vi "Test Display API.vi"() -> ()   [LabVIEW 2021]
doc: "Display API Tester."
uses:
  Display.lvlib
panel:
  out "ModuleName":string
  in  "Sim?":bool
  in  "Simulation":bool
  in  "Show Block Diagram":bool
  in  "Stop Module":bool
  in  "Start Module":bool
  in  "Hide Module Panel":bool
  in  "Show Module Panel":bool
  out "Status":string
  out "Module Running?":bool
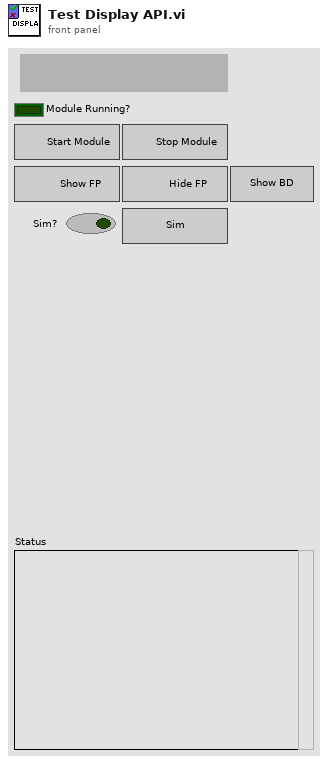
[diagram p1: front panel]
types:
  T1 = typedef "Display.lvlib/Broadcast Events--cluster.ctl" = cluster{"Module Did Init":refnum<user-event>, "Status Updated":refnum<user-event>, "Error Reported":refnum<user-event>, "Module Did Stop":refnum<user-event>, "Update Module Execution Status":refnum<user-event>}
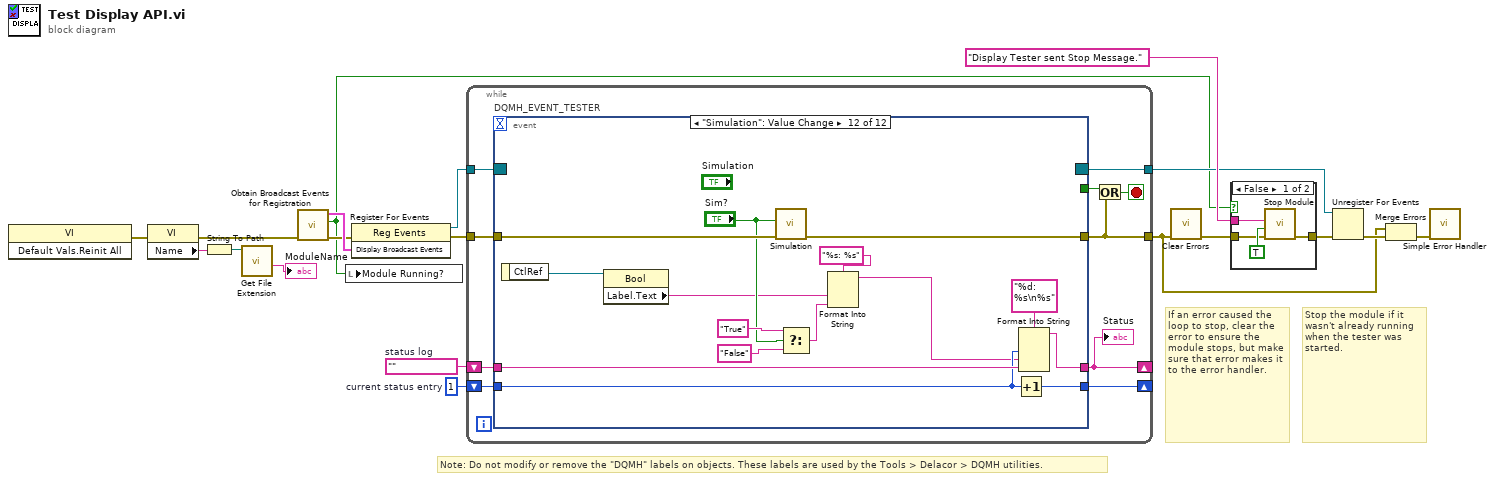
[diagram p0: block diagram]
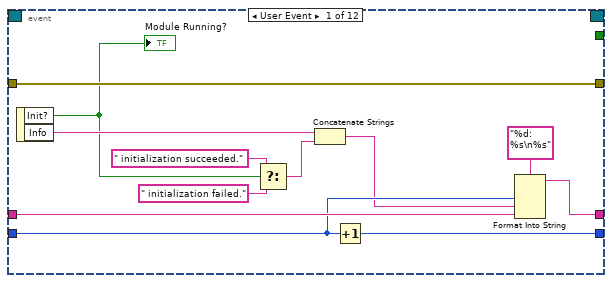
[diagram p3: hidden frame]
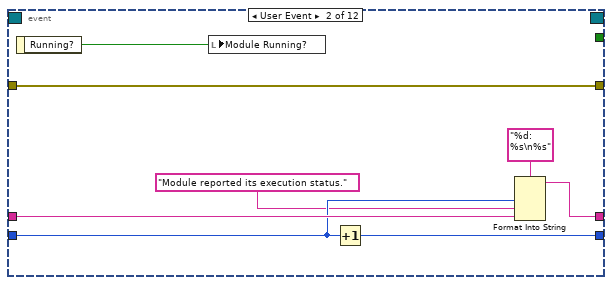
[diagram p4: hidden frame]
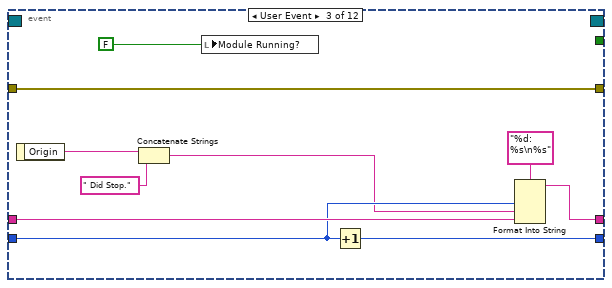
[diagram p5: hidden frame]
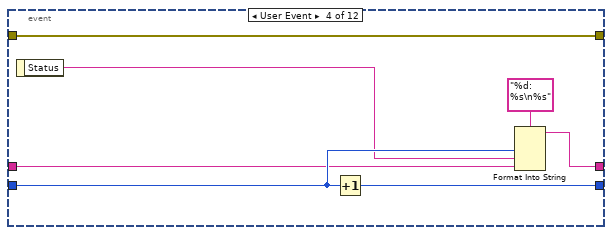
[diagram p6: hidden frame]
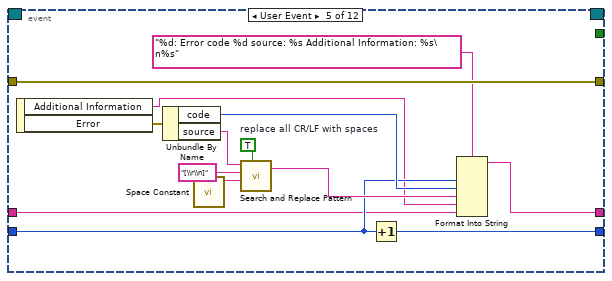
[diagram p7: hidden frame]
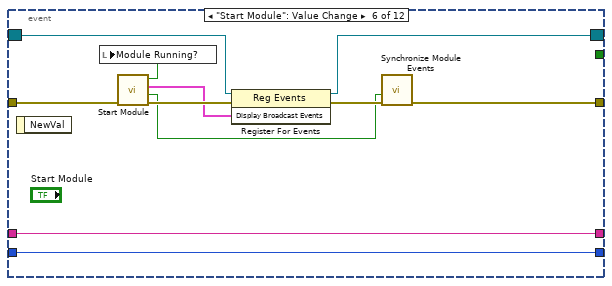
[diagram p8: hidden frame]
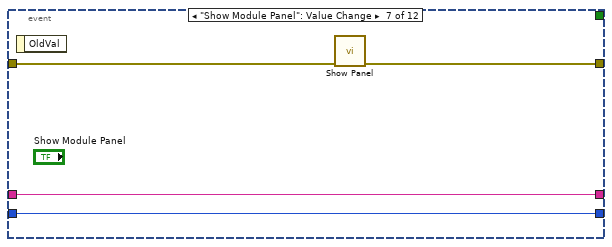
[diagram p9: hidden frame]
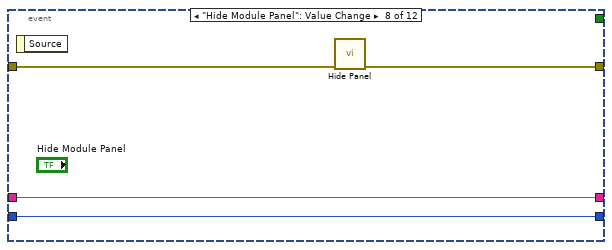
[diagram p10: hidden frame]
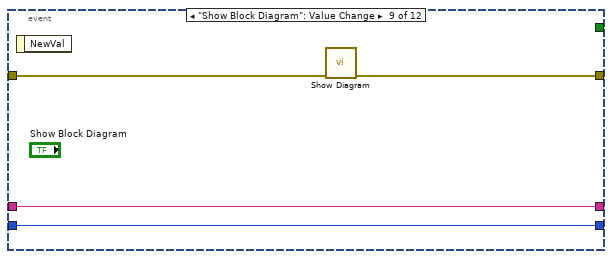
[diagram p11: hidden frame]
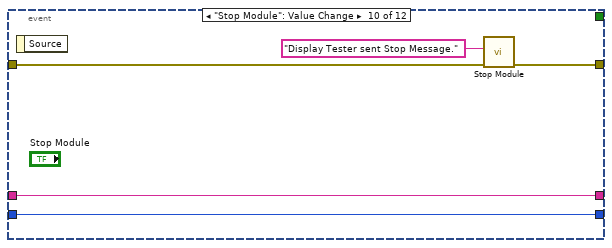
[diagram p12: hidden frame]
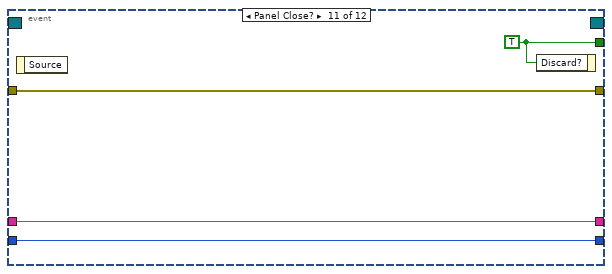
[diagram p13: hidden frame]
diagram:
  w15 = 1  # current status entry
  w16 = ""  # status log
  # "Stop the module if it wasn't already running when the tester was started."
  # "If an error caused the loop to stop, clear the error to ensure the module stops, but make sure that error makes it to the error handler."
  # "Note: Do not modify or remove the \"DQMH\" labels on objects. These labels are used by the Tools > Delacor > DQMH utilities."
  n1 = invoke class="VI" method="Default Vals.Reinit All"() -> (error out=w5:errorcluster)  [unwired: 3 in, 2 out]
  n2 = property class="VI"(error in=w5) -> (error out=w4:errorcluster, "Name"=w2:string)  [unwired: 1 in, 1 out]
  n3 = String To Path(string=w2) -> (path=w1:path)
  n4 = call <vilib>:"Get File Extension.vi"("file"=w1) -> ("filename without extension"=→"ModuleName":string)  [unwired: 6 in, 4 out]
  n5 = call "Obtain Broadcast Events for Registration.vi"("error in (no error)"=w4) -> ("error out"=w7:errorcluster, "Already running?"=w6:bool, "Display Broadcast Events"=w13:T1)  [unwired: 8 in]
  n6 = local write "Module Running?"(w6) -> ()
  n7 = register-events(error in=w7, w13) -> (reference out=w12:refnum<event-registration>, error out=w14:errorcluster)  [unwired: 1 in]
  n8 = while {
    tunnel: w12 -> [w29]
    tunnel: [w20] -> w8
    shift-right: [w24] -> _
    shift-left: w16 -> [w26]
    shift-right: [w25] -> _
    shift-left: w15 -> [w27]
    tunnel: w14 -> [w22]
    tunnel: [w21] -> w11
    stop <- w23 stop-if-true
    n9 = event "DQMH_EVENT_TESTER" shown="[11] \"Simulation\": Value Change" {
      selector: w29 -> [_ _ _ _ _ w85 _ _ _ _ _ _]
      dyn-events: [_ _ _ _ _ w84 _ _ _ _ _ _] -> w21
      timeout: _ -> [_ _ _ _ _ _ _ _ _ _ _ _]
      tunnel: [_ _ _ _ _ _ _ _ _ _ w112 _] -> w28
      tunnel: [w41 w43 w50 w60 w80 w83 w95 w99 w100 w106 w109 w126] -> w20
      tunnel: w27 -> [w38 w47 w57 w63 w70 w88 w93 w97 w101 w107 w110 w121]
      tunnel: w26 -> [w39 w48 w58 w62 w68 w89 w94 w98 w102 w108 w111 w124]
      tunnel: [w36 w45 w55 w64 w71 w89 w94 w98 w102 w108 w111 w123] -> w24
      tunnel: [w37 w46 w56 w66 w69 w88 w93 w97 w101 w107 w110 w122] -> w25
      tunnel: w22 -> [w41 w43 w50 w60 w80 w82 w92 w96 w103 w104 w109 w127]
      event User Event {
        n10 = event-data() -> ("Init?"=w33:bool, "Info"=w35:string)  [unwired: 1 in]
        "Module Running?" <- w33
        n11 = Select(t=" initialization succeeded.", s=w33, f=" initialization failed.") -> (s? t:f=w30:string)
        n12 = Concatenate Strings(w35, w30) -> (w34:string)
        n13 = Increment(x=w38) -> (x+1=w37:i32)
        n14 = Format Into String(format string="%d: %s\n%s", w38, w34, w39) -> (resulting string=w36:string)  [unwired: 2 in, 1 out]
      }
      event User Event {
        n15 = event-data() -> ("Running?"=w42:bool)  [unwired: 1 in]
        n16 = local write "Module Running?"(w42) -> ()
        n17 = Increment(x=w47) -> (x+1=w46:i32)
        n18 = Format Into String(format string="%d: %s\n%s", w47, "Module reported its execution status.", w48) -> (resulting string=w45:string)  [unwired: 2 in, 1 out]
      }
      event User Event {
        n19 = event-data() -> ("Origin"=w54:string)  [unwired: 1 in]
        n20 = Concatenate Strings(w54, " Did Stop.") -> (w53:string)
        n21 = local write "Module Running?"(FALSE ("Module Did Init?")) -> ()
        n22 = Increment(x=w57) -> (x+1=w56:i32)
        n23 = Format Into String(format string="%d: %s\n%s", w57, w53, w58) -> (resulting string=w55:string)  [unwired: 2 in, 1 out]
      }
      event User Event {
        n24 = event-data() -> ("Status"=w61:string)  [unwired: 1 in]
        n25 = Increment(x=w63) -> (x+1=w66:i32)
        n26 = Format Into String(format string="%d: %s\n%s", w63, w61, w62) -> (resulting string=w64:string)  [unwired: 2 in, 1 out]
      }
      event User Event {
        w76 = TRUE  # replace all CR/LF with spaces
        n27 = event-data() -> ("Additional Information"=w67:string, "Error"=w72:errorcluster)  [unwired: 1 in]
        n28 = Unbundle By Name(w72) -> ("code"=w73:i32, "source"=w74:string)
        n29 = call <vilib>:"Space Constant.vi"() -> ("String"=w77:string)
        n30 = call <vilib>:"Search and Replace Pattern.vi"("string"=w74, "regular expression (\"\")"="[\\r\\n]" ("regular expression (\"\")"), "replace string (\"\")"=w77, "replace all? (F)"=w76) -> ("result string"=w75:string)  [unwired: 1 in, 1 out]
        n31 = Increment(x=w70) -> (x+1=w69:i32)
        n32 = Format Into String(format string="%d: Error code %d source: %s Additional Information: %s\n%s", w70, w73, w75, w67, w68) -> (resulting string=w71:string)  [unwired: 2 in, 1 out]
      }
      event "Start Module": Value Change {
        n33 = event-data() -> ()  [unwired: 1 in, 1 out]
        n34 = call "Start Module.vi"("error in (no error)"=w82) -> ("error out"=w90:errorcluster, "Wait for Event Sync?"=w87:bool, "Display Broadcast Events"=w86:T1, "Module Was Already Running?"=w81:bool)  [unwired: 7 in]
        n35 = local write "Module Running?"(w81) -> ()
        n36 = register-events(reference=w85, error in=w90, w86) -> (reference out=w84:refnum<event-registration>, error out=w91:errorcluster)
        n37 = call "Synchronize Module Events.vi"("error in (no error)"=w91, "Wait for Event Sync?"=w87) -> ("error out"=w83:errorcluster)  [unwired: 9 in]
      }
      event "Show Module Panel": Value Change {
        n38 = event-data() -> ()  [unwired: 1 in, 1 out]
        n39 = call "Show Panel.vi"("error in (no error)"=w92) -> ("error out"=w95:errorcluster)  [unwired: 10 in]
      }
      event "Hide Module Panel": Value Change {
        n40 = event-data() -> ()  [unwired: 1 in, 1 out]
        n41 = call "Hide Panel.vi"("error in (no error)"=w96) -> ("error out"=w99:errorcluster)  [unwired: 10 in]
      }
      event "Show Block Diagram": Value Change {
        n42 = event-data() -> ()  [unwired: 1 in, 1 out]
        n43 = call "Show Diagram.vi"("error in (no error)"=w103) -> ("error out"=w100:errorcluster)  [unwired: 10 in]
      }
      event "Stop Module": Value Change {
        n44 = event-data() -> ()  [unwired: 1 in, 1 out]
        n45 = call "Stop Module.vi"("error in (no error)"=w104, "Origin"="Display Tester sent Stop Message.") -> ("error out"=w106:errorcluster)  [unwired: 9 in]
      }
      event Panel Close? {
        w112 = TRUE ("Discard?")
        n46 = event-data() -> ()  [unwired: 1 in, 1 out]
        n47 = event-data("Discard?"=w112) -> ()  [unwired: 1 in, 1 out]
      }
      event "Simulation": Value Change {
        n48 = event-data() -> ("CtlRef"=w120:refnum<vi>)  [unwired: 1 in]
        n49 = property class="Bool"(reference=w120) -> ("Label.Text"=w115:string)  [unwired: 1 in, 2 out]
        n50 = call "Simulation.vi"("error in (no error)"=w127, "Sim?"="Sim?") -> ("error out"=w126:errorcluster)  [unwired: 9 in]
        n51 = Select(t="True", s="Sim?", f="False") -> (s? t:f=w117:string)
        n52 = Format Into String(format string="%s: %s", w115, w117) -> (resulting string=w114:string)  [unwired: 2 in, 1 out]
        n53 = Increment(x=w121) -> (x+1=w122:i32)
        n54 = Format Into String(format string="%d: %s\n%s", w121, w114, w124) -> (resulting string=w123:string)  [unwired: 2 in, 1 out]
      }
    }
    "Status" <- w24
    n55 = Or(x=w28, y=w20) -> (x .or. y?=w23:bool)
  }
  n56 = call <vilib>:"Clear Errors.vi"("error in (no error)"=w8) -> ("error out"=w10:errorcluster)  [unwired: 5 in, 1 out]
  n57 = case shown="False" w6 {
    tunnel: [w131 w132] -> w18
    tunnel: "Display Tester sent Stop Message." ("Origin") -> [w130 _]
    tunnel: w10 -> [w128 w132]
    frame False {
      n58 = call "Stop Module.vi"("error in (no error)"=w128, "Wait for Module to Stop? (F)"=TRUE ("Wait for Module to stop?"), "Origin"=w130) -> ("error out"=w131:errorcluster)  [unwired: 8 in]
    }
    frame True {
    }
  }
  n59 = Unregister For Events(event registration refnum=w11, error in=w18) -> (error out=w19:errorcluster)
  n60 = Merge Errors(w8, w19) -> (w9:errorcluster)
  n61 = call <vilib>:"Simple Error Handler.vi"("error in (no error)"=w9) -> ()  [unwired: 4 in, 5 out]
